vi "TestRFGVBedURL.vi"(9 "BedURL":string="192.168.0.1", 10 "FGV Room":i32=102) -> (2 "Pass":bool)   [LabVIEW 2015]
uses:
  TypeDef/RoomsActionEnum.ctl
panel:
  out "JSON string":string
  out "Read 2":string
  out "Read1":string
  out "Write":string
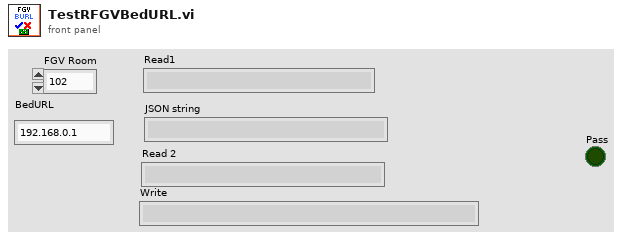
[diagram p1: front panel]
types:
  T1 = typedef "RoomsActionEnum.ctl" = enum16{"Init", "Add Room", "Remove Room", "Read Room", "Read Flag", "Read Flag State", "Write Flag State", "Read Flag Color", "Write Flag Color", "Read Bed Vacant", "Write Bed Vacant", "Read Personnel", "Add Personnel", "Remove Personnel", "Read Requests", "Add Request", "Remove Request", "Read Beacon ID", "Write Beacon ID", "Write Bed URL", "Read Bed URL", "Read Rooms Numbers", "Write Flag"}
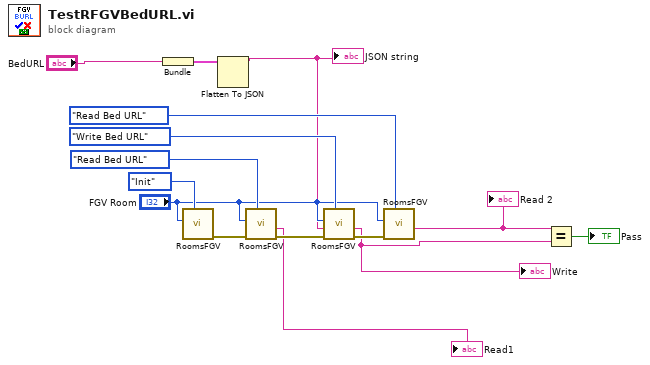
[diagram p0: block diagram]
diagram:
  n1 = Bundle("BedURL"="BedURL") -> (w4:cluster{"BedURL":string})  [unwired: 1 in]
  n2 = call "RoomsFGV.vi"("Actions"=RoomsActionEnum."Init", "Room"="FGV Room") -> ("error out"=w14:errorcluster)  [unwired: 8 in, 1 out]
  n3 = Flatten To JSON(anything=w4) -> (JSON string=w3:string)  [unwired: 2 in, 1 out]
  "JSON string" <- w3
  n4 = call "RoomsFGV.vi"("Actions"=RoomsActionEnum."Read Bed URL", "error in (no error)"=w14, "Room"="FGV Room") -> ("error out"=w13:errorcluster, "Data Out"=→"Read1":string)  [unwired: 7 in]
  n5 = call "RoomsFGV.vi"("Actions"=RoomsActionEnum."Write Bed URL", "error in (no error)"=w13, "Data In"=w3, "Room"="FGV Room") -> ("error out"=w12:errorcluster, "Data Out"=w1:string)  [unwired: 6 in]
  "Write" <- w1
  n6 = call "RoomsFGV.vi"("Actions"=RoomsActionEnum."Read Bed URL", "error in (no error)"=w12, "Room"="FGV Room") -> ("Data Out"=w2:string)  [unwired: 7 in, 1 out]
  "Read 2" <- w2
  n7 = Equal?(x=w2, y=w1) -> (x = y?=→"Pass":bool)
